vi "EVAL.vi"(0 "TCP session in":refnum<k5>, 5 "lua script":string, 7 "KEYS":string[](array[string]), 9 "ARGV":string[](array[string]), 11 "error in":errorcluster) -> (4 "TCP session out":refnum<k5>, 6 "Data":T1, 8 "string data":string[](array[string]), 15 "error out":errorcluster)   [LabVIEW 2023]
uses:
  SubVIs/Controls/redis-data.ctl
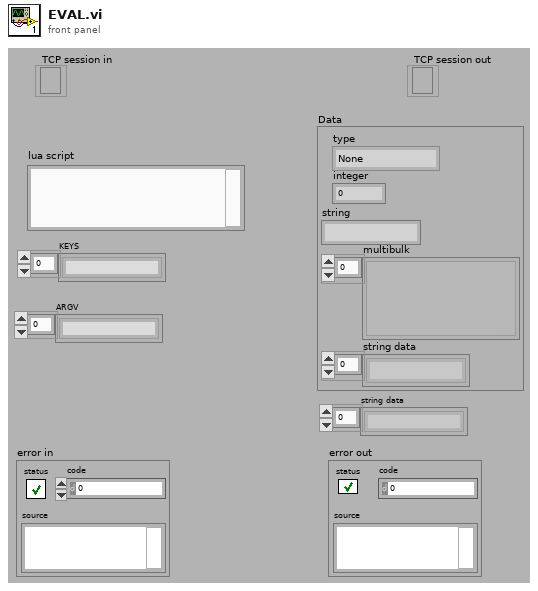
[diagram p1: front panel]
types:
  T1 = typedef "redis-data.ctl" = cluster{"type":enum16{"None", "Error", "Status", "Nil", "Integer", "String", "Multibulk"}, "integer":i64, "string":string, "multibulk":variant[], "string data":string[]}
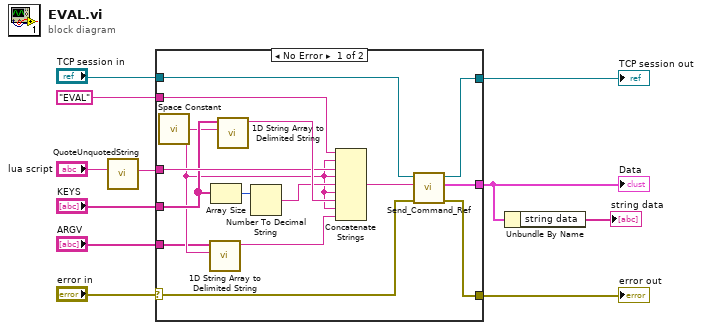
[diagram p0: block diagram]
diagram:
  n1 = call "QuoteUnquotedString.vi"("String in"="lua script") -> ("String out"=w1:string)  [unwired: 10 in]
  n2 = case shown="No Error" "error in" {
    selector: "error in" -> [w26 w28]
    tunnel: w1 -> [w16 _]
    tunnel: "EVAL" -> [w17 _]
    tunnel: "TCP session in" -> [w23 w27]
    tunnel: [w25 w28] -> w9
    tunnel: [w24 _] -> w4
    tunnel: [w22 w27] -> w7
    tunnel: "KEYS" -> [w15 _]
    tunnel: "ARGV" -> [w13 _]
    frame No Error {
      n3 = call <vilib>:"Space Constant.vi"() -> ("String"=w14:string)
      n4 = call <vilib>:"1D String Array to Delimited String.vi"("delimiter"=w14, "string array"=w13) -> ("delimited string"=w12:string)  [unwired: 9 in]
      n5 = Array Size(array=w15) -> (size(s)=w19:i32)
      n6 = call <vilib>:"1D String Array to Delimited String.vi"("delimiter"=w14, "string array"=w15) -> ("delimited string"=w21:string)  [unwired: 9 in]
      n7 = Number To Decimal String(number=w19) -> (decimal integer string=w20:string)  [unwired: 1 in]
      n8 = Concatenate Strings(w17, w14, w16, w14, w20, w14, w21, w14, w12) -> (w18:string)
      n9 = call "Send_Command_Ref.vi"("error in"=w26, "command"=w18, "TCP session in"=w23) -> ("error out"=w25:errorcluster, "Data"=w24:T1, "TCP session out"=w22:refnum<k5>)  [unwired: 6 in]
    }
    frame Error {
    }
  }
  "error out" <- w9
  "TCP session out" <- w7
  "Data" <- w4
  n10 = Unbundle By Name(w4) -> ("string data"=→"string data":string[])
